vi "JJMCclase 6.vi"() -> ()   [LabVIEW 2011]
panel:
  out "ALARMA":bool
  out "Temperatura":dbl(slide) scale=0.0..100.0
  out "Velocidad Super Rapida":bool
  out "Velocidad Rapida":bool
  out "Velocidad Lenta":bool
  out "velocidad":i32(knob) scale=0.0..220.0
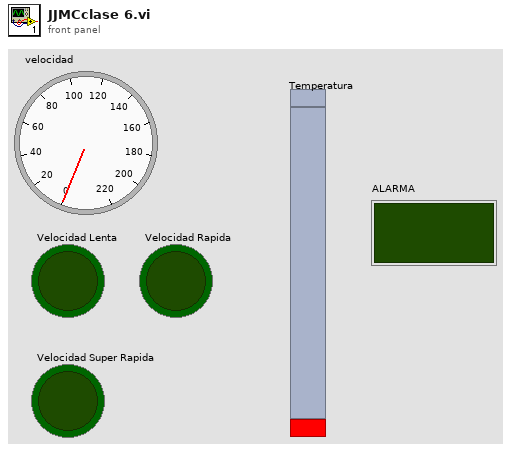
[diagram p1: front panel]
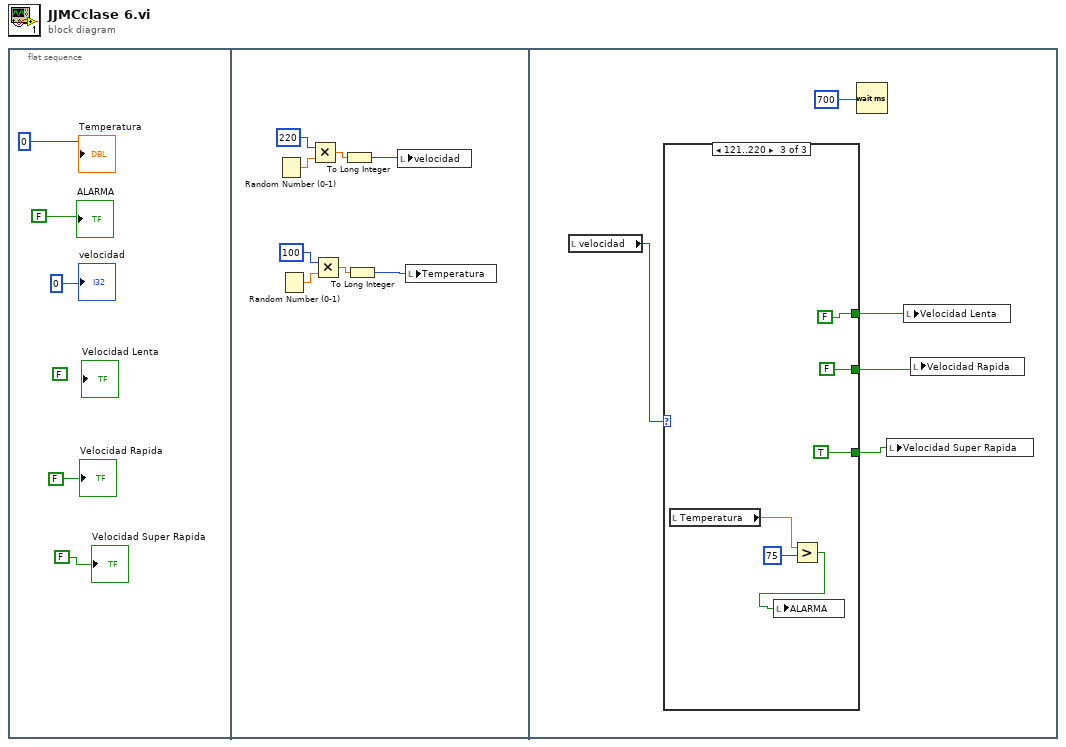
[diagram p0: block diagram]
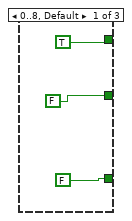
[diagram p2: hidden frame]
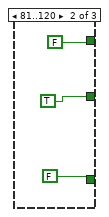
[diagram p3: hidden frame]
diagram:
  n1 = flat-sequence {
    frame #0 {
      (unwired) FALSE
      "Velocidad Rapida" <- FALSE
      "Temperatura" <- 0
      "ALARMA" <- FALSE
      "Velocidad Super Rapida" <- FALSE
      "velocidad" <- 0
    }
    frame #1 {
      n2 = Random Number (0-1)() -> (number: 0 to 1=w12:dbl)
      n3 = Random Number (0-1)() -> (number: 0 to 1=w8:dbl)
      n4 = Multiply(x=220, y=w12) -> (x*y=w10:dbl)
      n5 = Multiply(x=100, y=w8) -> (x*y=w9:dbl)
      n6 = To Long Integer(number=w10) -> (32bit integer=w11:i32)
      n7 = To Long Integer(number=w9) -> (32bit integer=w6:i32)
      n8 = local write "velocidad"(w11) -> ()
      n9 = local write "Temperatura"(w6) -> ()
    }
    frame #2 {
      n10 = local read "velocidad"() -> (w18:i32)
      n11 = case shown="121..220" w18 {
        tunnel: [FALSE FALSE TRUE] -> w17
        tunnel: [TRUE FALSE FALSE] -> w16
        tunnel: [FALSE TRUE FALSE] -> w15
        frame 0..8, Default {
        }
        frame 81..120 {
        }
        frame 121..220 {
          n12 = local read "Temperatura"() -> (w26:dbl)
          n13 = Greater?(x=w26, y=75) -> (0:w25:bool)
          n14 = local write "ALARMA"(w25) -> ()
        }
      }
      n15 = Wait (ms)(milliseconds to wait=700) -> ()  [unwired: 1 out]
      n16 = local write "Velocidad Super Rapida"(w17) -> ()
      n17 = local write "Velocidad Lenta"(w16) -> ()
      n18 = local write "Velocidad Rapida"(w15) -> ()
    }
  }
